vi "HW_6p1_Task2_PRADHASK.vi"() -> ()   [LabVIEW 2016]
uses:
  <vilib>/express/express arith-compare/Formula/XNode/ExpressFormulaBlockNode.xnode
panel:
  in  "Connection Type":string
  out "Ktotal":dbl
  in  "K2":dbl
  in  "K1":dbl
  # "Write in lower case (series/ parallel)"
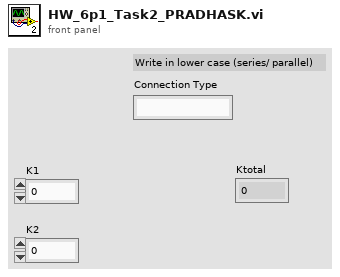
[diagram p1: front panel]
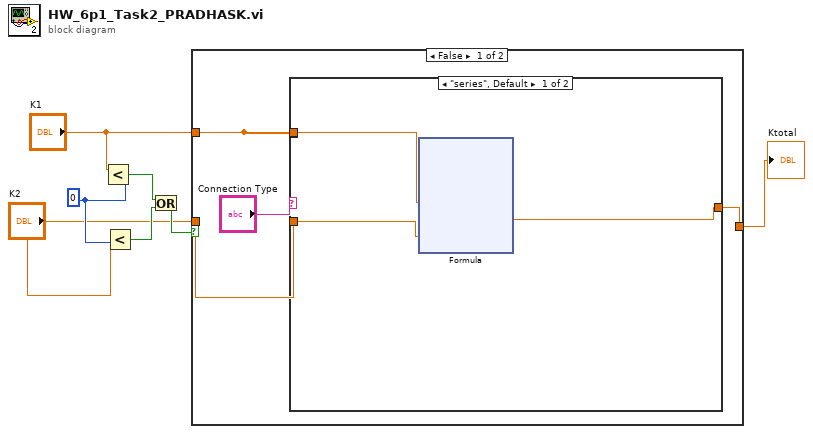
[diagram p0: block diagram]
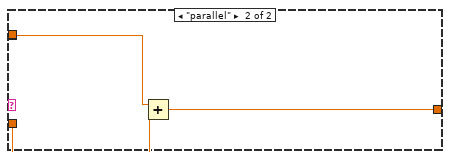
[diagram p2: hidden frame]
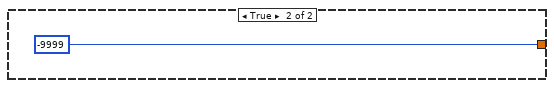
[diagram p3: hidden frame]
diagram:
  w7 = 0
  n1 = Less?(x="K1", y=w7) -> (x < y?=w6:bool)
  n2 = Less?(x="K2", y=w7) -> (x < y?=w5:bool)
  n3 = Or(x=w6, y=w5) -> (x .or. y?=w4:bool)
  n4 = case shown="False" w4 {
    tunnel: [w10 -9999] -> w3
    tunnel: "K1" -> [w9 _]
    tunnel: "K2" -> [w8 _]
    frame False {
      n5 = case shown="\"series\", Default" "Connection Type" {
        tunnel: w9 -> [_ w27]
        tunnel: [w12 w25] -> w10
        tunnel: w9 -> [w14 _]
        tunnel: w8 -> [w13 w26]
        frame "series", Default {
          n6 = xnode "Formula"("K1"=w14, "K2"=w13) -> ("Result"=w12:dbl)  [unwired: 1 in, 1 out]
        }
        frame "parallel" {
          n7 = Add(x=w27, y=w26) -> (x+y=w25:dbl)
        }
      }
    }
    frame True {
    }
  }
  "Ktotal" <- w3
